vi "Simulate Data.vi"() -> ()   [LabVIEW 2010]
doc: "This VI simulates data acquisition using both a For Loop and a While Loop and compares the results."
panel:
  out "Equivalent Output?":bool
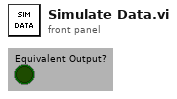
[diagram p1: front panel]
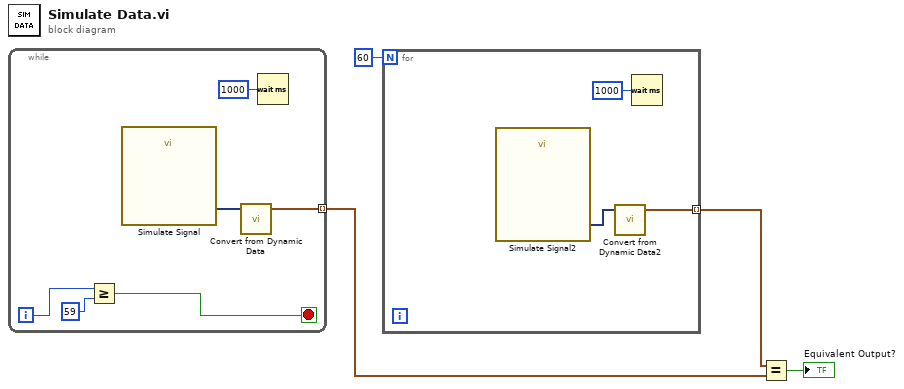
[diagram p0: block diagram]
diagram:
  n1 = while {
    tunnel: [w5] -> w2 mode=indexing
    i -> [w9]
    stop <- w7 stop-if-true
    n2 = Greater Or Equal?(x=w9, y=59) -> (x >= y?=w7:bool)
    n3 = call "Simulate Signal"() -> ("Sine"=w6:dynamicdata)  [unwired: 14 in, 1 out]
    n4 = call "Convert from Dynamic Data"("Dynamic Data Type"=w6) -> ("Waveform"=w5:waveform(dbl))  [unwired: 3 in]
    n5 = Wait (ms)(milliseconds to wait=u32 1000) -> ()  [unwired: 1 out]
  }
  n6 = for {
    N: 60 ("y") -> [_]
    tunnel: [w11] -> w3 mode=indexing
    n7 = call "Simulate Signal2"() -> ("Sine"=w12:dynamicdata)  [unwired: 14 in, 1 out]
    n8 = call "Convert from Dynamic Data2"("Dynamic Data Type"=w12) -> ("Waveform"=w11:waveform(dbl))  [unwired: 3 in]
    n9 = Wait (ms)(milliseconds to wait=u32 1000) -> ()  [unwired: 1 out]
  }
  n10 = Equal?(x=w3, y=w2) -> (x = y?=→"Equivalent Output?":bool)
